vi "Plot Helper (Vector).vi"(8 "error in (no error)":errorcluster, 9 "radius vector":dbl[](array[numeric]), 10 "theta vector":dbl[](array[numeric]), 11 "2D Plot Class Obj Array in":refnum<class "2D Plot Datatype.lvclass">[](array[class])) -> (0 "error out":errorcluster, 3 "2D Plot Class Obj Array out":refnum<class "2D Plot Datatype.lvclass">[](array[class]))   [LabVIEW 2017, in "2D Compass Datatype.lvclass"]
doc: "Graphs vectors that emanate from the center origin in a compass plot. Multiple references to this VI generate multiple plots on the same graph."
uses:
  <vilib>/Math Plots/2D Math Plots/2D Compass/2D Compass Datatype/2D Compass Datatype.lvclass
  <vilib>/Math Plots/2D Math Plots/2D Plot/2D Plot Datatype/2D Plot Datatype.lvclass
  e:/builds/penguin/labview/branches/2017/dev/dist/vi.lib/Math Plots/2D Math Plots/2D Plot/2D Plot Datatype/2D Plot Datatype.lvclass
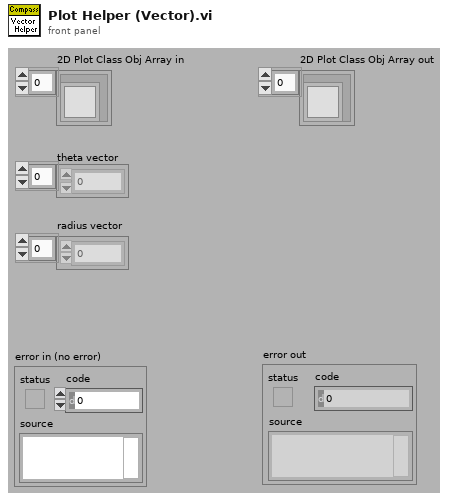
[diagram p1: front panel]
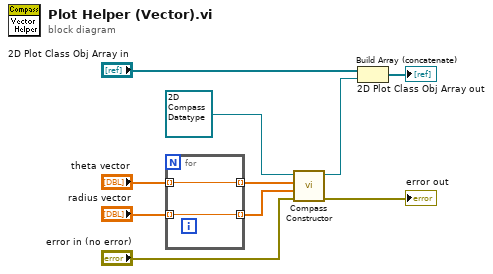
[diagram p0: block diagram]
diagram:
  n1 = for {
    tunnel: [w12] -> w4 mode=indexing
    tunnel: "theta vector" -> [w12] mode=indexing
    tunnel: [w11] -> w2 mode=indexing
    tunnel: "radius vector" -> [w11] mode=indexing
  }
  n2 = call <vilib>:"Compass Constructor.vi"("error in (no error)"="error in (no error)", "radius vector"=w2, "theta vector"=w4, "2D Compass Datatype.lvclass in"=refnum<class "2D Compass Datatype.lvclass"> refnum ("3D Quiver Datatype.lvclass in")) -> ("error out"=→"error out":errorcluster, "2D Compass Datatype.lvclass out"=w6:refnum<class "2D Compass Datatype.lvclass">)  [unwired: 1 in, 5 out]
  n3 = Build Array (concatenate)("2D Plot Class Obj Array in", w6) -> (→"2D Plot Class Obj Array out":refnum<class "2D Plot Datatype.lvclass">[])
